vi "BoP Input Read Client.vi"() -> ()   [LabVIEW 2017]
uses:
  <vilib>/OPCUA/controls/NodeIds.ctl
  <vilib>/OPCUA/controls/NodeId.ctl
  <vilib>/OPCUA/NI OPC UA Client.lvlib
panel:
  in  "stop":bool
  out "error out":errorcluster
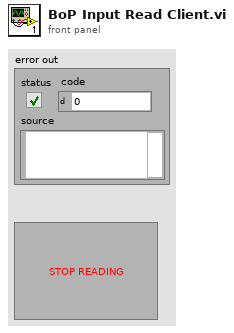
[diagram p1: front panel]
types:
  T1 = cluster{"message mode":enum16{"None", "Sign", "Sign and Encrypt"}, "security":enum16{"Basic256", "Basic128Rsa15"}}
  T2 = typedef "NodeIds.ctl" = T3[]
  T3 = typedef "NodeId.ctl" = string
  T4 = typedef "OPC UA Client Refnum.ctl" = refnum<k21>
  T5 = typedef "Subscription ID.ctl" = u32
  T6 = typedef "Subscription Data Change.ctl" = cluster{"node ID":T3, " value":variant, "timestamp":timestamp, "data type":T7, "status code":T8}
  T7 = typedef "Data Type.ctl" = u16
  T8 = typedef "OPC UA StatusCode.ctl" = u32
  T9 = cluster{"[0]":sgl, "[1]":sgl, "[2]":sgl, "[3]":sgl, "[4]":sgl, "[5]":sgl, "[6]":sgl, "[7]":sgl, "[8]":sgl, "[9]":sgl, "[10]":sgl}
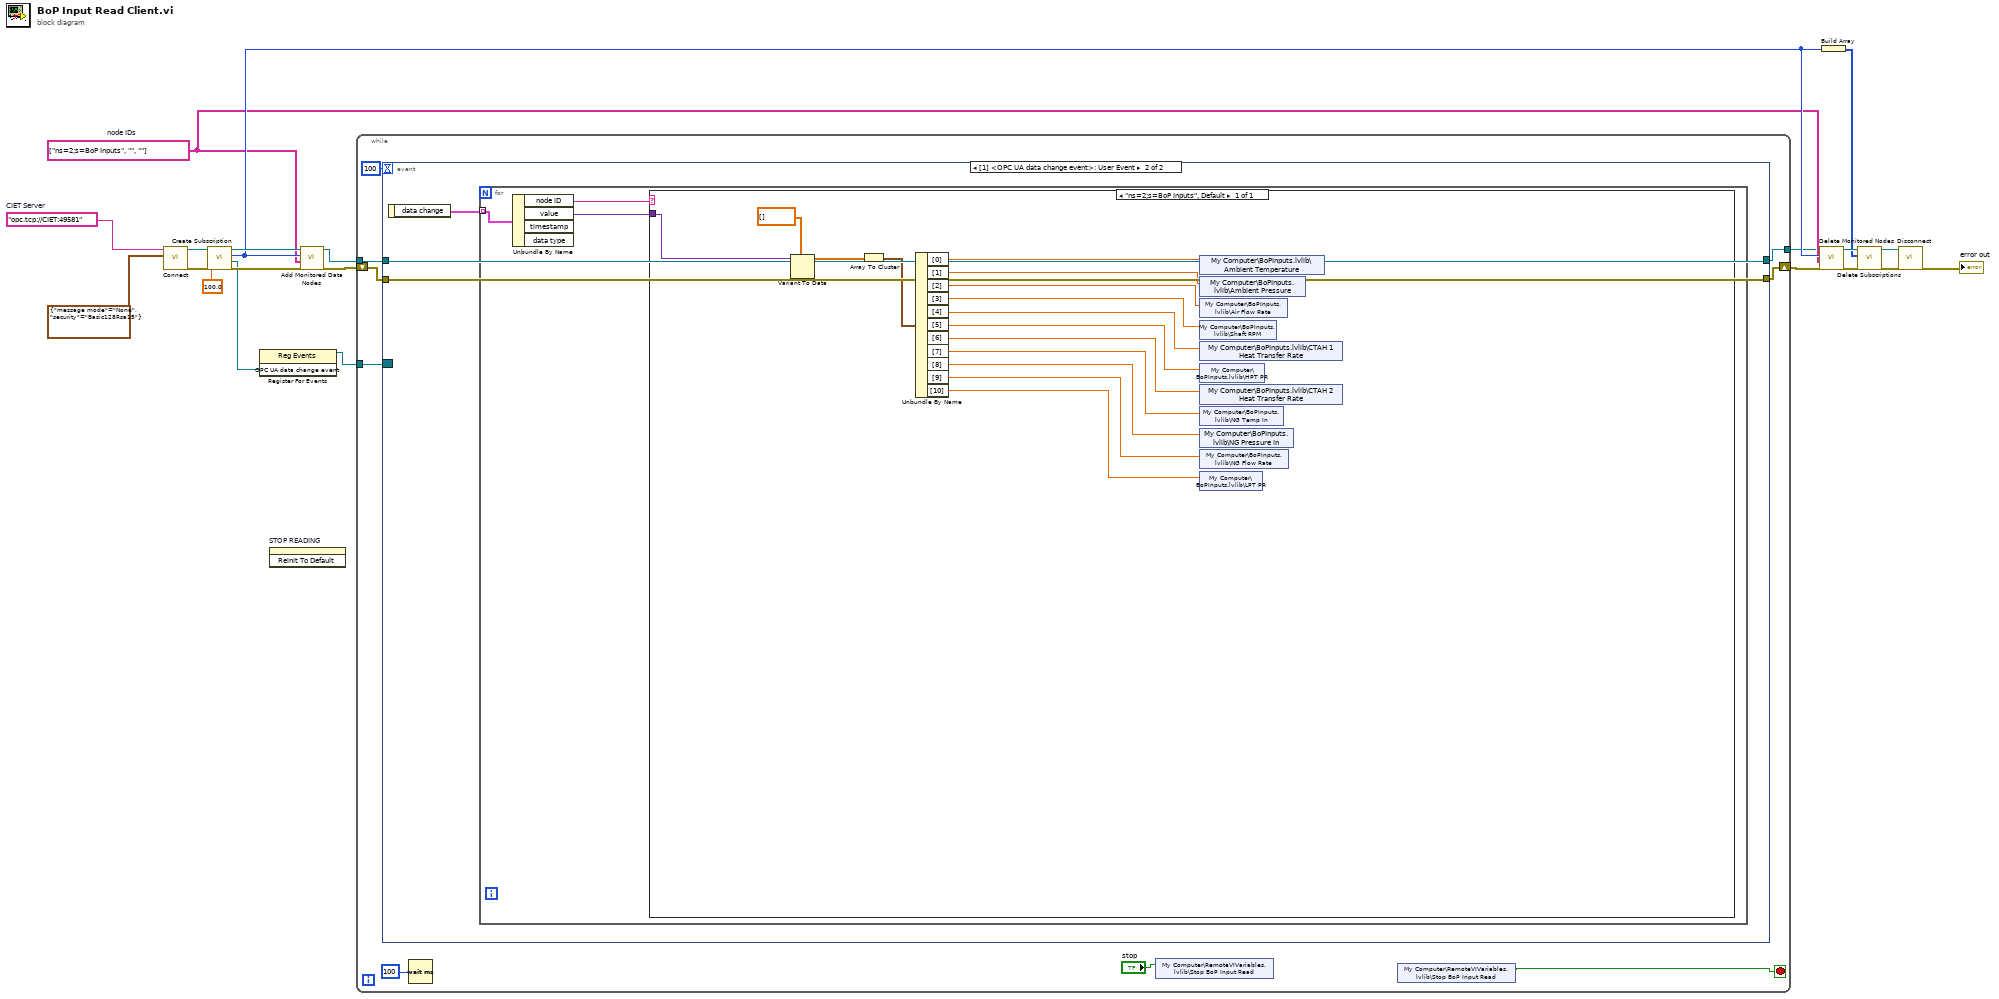
[diagram p0: block diagram]
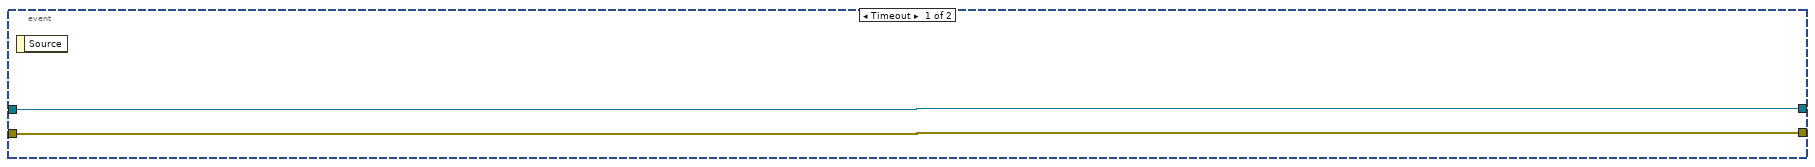
[diagram p2: hidden frame]
diagram:
  w5 = T2 ["ns=2;s=BoP Inputs", "", ""]  # node IDs
  w20 = "opc.tcp://CIET:49581"  # CIET Server
  n1 = call <vilib>:"Connect.vi"("security policy"=T1 {"message mode"=enum."None", "security"=enum."Basic128Rsa15"}, "server endpoint URL"=w20) -> ("error out"=w2:errorcluster, "OPC UA client refnum out"=w18:T4)  [unwired: 7 in, 1 out]
  n2 = call <vilib>:"Create Subscription.vi"("error in (no error)"=w2, "publishing interval (1000 ms)"=100.0, "OPC UA client refnum in"=w18) -> ("error out"=w16:errorcluster, "OPC UA data change event"=w15:refnum<user-event>, "subscription ID out"=w10:T5, "OPC UA client refnum out"=w17:T4)  [unwired: 4 in, 1 out]
  n3 = register-events(w15) -> (reference out=w8:refnum<event-registration>)  [unwired: 2 in, 1 out]
  n4 = invoke on="STOP READING" class="Bool" method="Reinit To Default"() -> ()  [unwired: 3 in, 3 out]
  n5 = call <vilib>:"Add Monitored Data Nodes.vi"("error in (no error)"=w16, "node IDs"=w5, "subscription ID in"=w10, "OPC UA client refnum in"=w17) -> ("error out"=w6:errorcluster, "OPC UA client refnum out"=w7:T4)  [unwired: 4 in, 2 out]
  n6 = while {
    tunnel: w8 -> [w30]
    tunnel: w7 -> [w29]
    tunnel: [w28] -> w4
    shift-right: [w26] -> w1
    shift-left: w6 -> [w25]
    stop <- w23 stop-if-true
    n7 = event shown="[1] <OPC UA data change event>: User Event" {
      selector: w30 -> [_ _]
      dyn-events: _ -> [_ _]
      timeout: 100 -> [_ _]
      tunnel: w29 -> [w32 w35]
      tunnel: [w32 w35] -> w28
      tunnel: w25 -> [w31 w34]
      tunnel: [w31 w34] -> w26
      event Timeout {
        n8 = event-data() -> ()  [unwired: 1 in, 1 out]
      }
      event User Event {
        n9 = event-data() -> ("data change"=w33:T6[])  [unwired: 1 in]
        n10 = for {
          tunnel: w33 -> [w38] mode=indexing
          n11 = Unbundle By Name(w38) -> ("node ID"=w37:T3, "value"=w36:variant)  [unwired: 2 out]
          n12 = case shown="\"ns=2;s=BoP Inputs\", Default" w37 {
            tunnel: w36 -> [w50]
            frame "ns=2;s=BoP Inputs", Default {
              n13 = Variant To Data(type=sgl[] [], Variant=w50) -> (data=w52:sgl[])  [unwired: 1 in, 1 out]
              n14 = Array To Cluster(array=w52) -> (cluster=w51:T9)
              n15 = Unbundle By Name(w51) -> ("[0]"=w49:sgl, "[1]"=w48:sgl, "[2]"=w47:sgl, "[3]"=w46:sgl, "[4]"=w45:sgl, "[5]"=w44:sgl, "[6]"=w43:sgl, "[7]"=w42:sgl, "[8]"=w41:sgl, "[9]"=w40:sgl, "[10]"=w39:sgl)
              n16 = shared-variable "My Computer\\BoPInputs.lvlib\\Ambient Temperature"(w49) -> ()  [unwired: 1 in, 1 out]
              n17 = shared-variable "My Computer\\BoPInputs.lvlib\\Ambient Pressure"(w48) -> ()  [unwired: 1 in, 1 out]
              n18 = shared-variable "My Computer\\BoPInputs.lvlib\\Air Flow Rate"(w47) -> ()  [unwired: 1 in, 1 out]
              n19 = shared-variable "My Computer\\BoPInputs.lvlib\\Shaft RPM"(w46) -> ()  [unwired: 1 in, 1 out]
              n20 = shared-variable "My Computer\\BoPInputs.lvlib\\CTAH 1 Heat Transfer Rate"(w45) -> ()  [unwired: 1 in, 1 out]
              n21 = shared-variable "My Computer\\BoPInputs.lvlib\\HPT PR"(w44) -> ()  [unwired: 1 in, 1 out]
              n22 = shared-variable "My Computer\\BoPInputs.lvlib\\CTAH 2 Heat Transfer Rate"(w43) -> ()  [unwired: 1 in, 1 out]
              n23 = shared-variable "My Computer\\BoPInputs.lvlib\\NG Temp In"(w42) -> ()  [unwired: 1 in, 1 out]
              n24 = shared-variable "My Computer\\BoPInputs.lvlib\\NG Pressure In"(w41) -> ()  [unwired: 1 in, 1 out]
              n25 = shared-variable "My Computer\\BoPInputs.lvlib\\NG Flow Rate"(w40) -> ()  [unwired: 1 in, 1 out]
              n26 = shared-variable "My Computer\\BoPInputs.lvlib\\LPT PR"(w39) -> ()  [unwired: 1 in, 1 out]
            }
          }
        }
      }
    }
    n27 = Wait (ms)(milliseconds to wait=u32 100 ("millisecond timer value")) -> ()  [unwired: 1 out]
    n28 = shared-variable "My Computer\\RemoteVIVariables.lvlib\\Stop BoP Input Read"("stop") -> ()  [unwired: 1 in, 1 out]
    n29 = shared-variable "My Computer\\RemoteVIVariables.lvlib\\Stop BoP Input Read"() -> (w23:bool)  [unwired: 1 in, 1 out]
  }
  n30 = call <vilib>:"Delete Monitored Nodes.vi"("error in (no error)"=w1, "node IDs"=w5, "subscription ID in"=w10, "OPC UA client refnum in"=w4) -> ("error out"=w11:errorcluster, "OPC UA client refnum out"=w12:T4)  [unwired: 3 in, 3 out]
  n31 = Build Array(w10) -> (w9:T5[])
  n32 = call <vilib>:"Delete Subscriptions.vi"("error in (no error)"=w11, "subscription IDs"=w9, "OPC UA client refnum in"=w12) -> ("error out"=w13:errorcluster, "OPC UA client refnum out"=w14:T4)  [unwired: 6 in, 1 out]
  n33 = call <vilib>:"Disconnect.vi"("error in (no error)"=w13, "OPC UA client refnum in"=w14) -> ("error out"=→"error out":errorcluster)  [unwired: 9 in]
